vi "test.vi"() -> ()   [LabVIEW 2023]
uses:
  Configurations/Read Write CFG/Red-y Read Write CFG.lvclass
  D:/git/HAL/HAL GOOP4/Configuration/Configuration JSON/Configuration JSON Base/CFG JSON.lvclass
  Configurations/Read Write CFG/Read Write PE Input.ctl
  Configuration/Configuration JSON/Configuration JSON Base/CFG JSON.lvclass
panel:
  out "Output":variant
  in  "error in":errorcluster
  out "error out":errorcluster
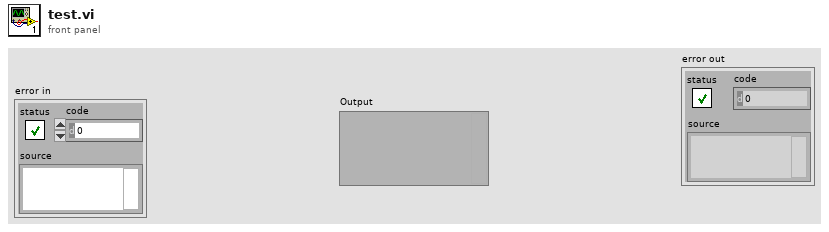
[diagram p1: front panel]
types:
  T1 = typedef "Read Write PE Input.ctl" = cluster{"Action":enum16{"Write", "Read"}, "Register Start Address":u16, "Data (Type)":variant}
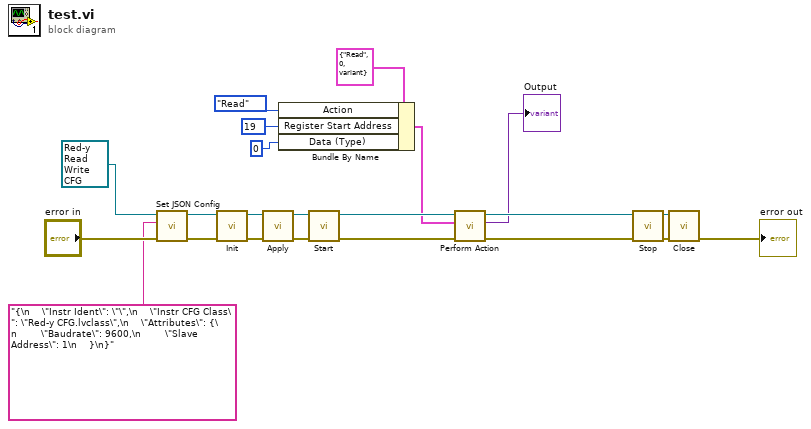
[diagram p0: block diagram]
diagram:
  n1 = call "Set JSON Config.vi"("error in (no error)"="error in", "<JSON>Config>"="{\n    \"Instr Ident\": \"\",\n    \"Instr CFG Class\": \"Red-y CFG.lvclass\",\n    \"Attributes\": {\n        \"Baudrate\": 9600,\n        \"Slave Address\": 1\n    }\n}", "CFG Base in"=refnum<class "Red-y Read Write CFG.lvclass"> refnum) -> ("error out"=w20:errorcluster, "CFG Base out"=w18:refnum<class "Red-y Read Write CFG.lvclass">)  [unwired: 7 in]
  n2 = call-dynamic "Init.vi"("error in"=w20, "CFG Base in"=w18) -> ("error out"=w22:errorcluster, "CFG Base out"=w3:refnum<class "Red-y Read Write CFG.lvclass">)  [unwired: 8 in]
  n3 = call-dynamic "Apply.vi"("error in"=w22, "Red-y Read Write CFG in"=w3) -> ("error out"=w4:errorcluster, "Red-y Read Write CFG out"=w2:refnum<class "Red-y Read Write CFG.lvclass">)  [unwired: 8 in]
  n4 = Bundle By Name(cluster=T1 {"Action"=enum."Read", "Register Start Address"=0, "Data (Type)"=variant}, "Action"=enum16{"Write", "Read"}."Read", "Register Start Address"=u16 19, "Data (Type)"=u16 0) -> (w6:T1)
  n5 = call-dynamic "Start.vi"("error in"=w4, "Red-y Read Write CFG in"=w2) -> ("error out"=w15:errorcluster, "Red-y Read Write CFG out"=w11:refnum<class "Red-y Read Write CFG.lvclass">)  [unwired: 8 in]
  n6 = call-dynamic "Perform Action.vi"("error in"=w15, "Input"=w6, "Red-y Read Write CFG in"=w11) -> ("error out"=w12:errorcluster, "Output"=→"Output":variant, "Red-y Read Write CFG out"=w10:refnum<class "Red-y Read Write CFG.lvclass">)  [unwired: 6 in]
  n7 = call-dynamic "Stop.vi"("error in"=w12, "Red-y Read Write CFG in"=w10) -> ("error out"=w14:errorcluster, "Red-y Read Write CFG out"=w13:refnum<class "Red-y Read Write CFG.lvclass">)  [unwired: 8 in]
  n8 = call-dynamic "Close.vi"("error in"=w14, "Red-y Read Write CFG in"=w13) -> ("error out"=→"error out":errorcluster)  [unwired: 8 in, 1 out]
